vi "PDLM_SetLHTargetTemp.vi"(8 "error in (no error)":errorcluster, 9 "TargTemp":sgl, 10 "ScaleID":T1, 11 "USBIdx":i32) -> (0 "error out":errorcluster, 3 "return type":i32)   [LabVIEW 2017]
uses:
  PDLM_ScaleID.ctl
  PDLM_DllPath_global.vi
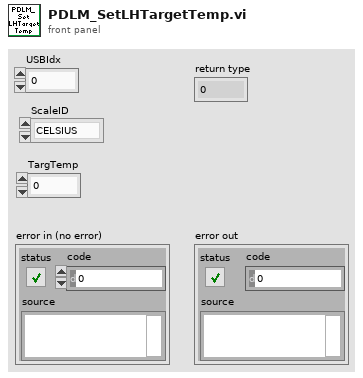
[diagram p1: front panel]
types:
  T1 = typedef "PDLM_ScaleID.ctl" = enum32{"CELSIUS", "FAHRENHEIT", "KELVIN"}
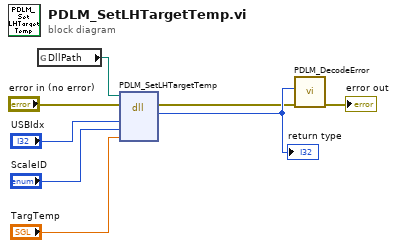
[diagram p0: block diagram]
diagram:
  n1 = global read "PDLM_DllPath_global.vi" "DllPath"() -> (w4:path)
  n2 = dll-call lib="M:/_dev/progs/LabVIEW/_lib/PQ/Taiko/pdlm_lib.dll" fn="PDLM_SetLHTargetTemp"(path in=w4, error in="error in (no error)", "USBIdx"="USBIdx", "ScaleID"="ScaleID", "TargTemp"="TargTemp") -> (error out=w6:errorcluster, "return type"=w7:i32)  [unwired: 4 in, 1 out]
  "return type" <- w7
  n3 = call "PDLM_DecodeError.vi"("error in (no error)"=w6, "code"=w7) -> ("error out"=→"error out":errorcluster)  [unwired: 7 in, 2 out]
